vi "Determine Path Points.vi"(8 "error in (no error)":errorcluster, 11 "Tool Path in":refnum<class "Tool Path.lvclass">) -> (0 "error out":errorcluster, 2 "Points":T1[](array[typedef]), 3 "Tool Path out":refnum<class "Tool Path.lvclass">)   [LabVIEW 2019, in "Tool Path.lvclass"]
uses:
  Tool Path.lvclass
  Parse/PathCommands/Point.ctl
  Parse/ParsePaths/Path.lvclass/Path.ctl
  Settings/Path Settings/Path Settings.lvclass/Path Settings.ctl
  Parse/PathCommands/PathCommands.lvclass
  Parse/ParsePaths/Path.lvclass
  Settings/Path Settings/Path Settings.lvclass
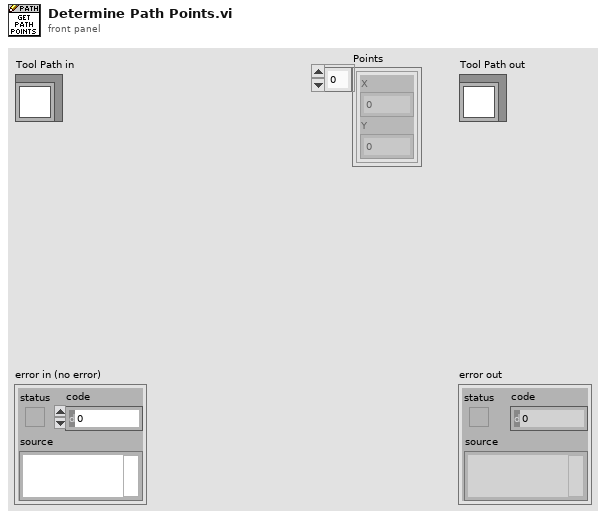
[diagram p1: front panel]
types:
  T1 = typedef "PathCommands.lvclass/Point.ctl" = cluster{"X":dbl, "Y":dbl}
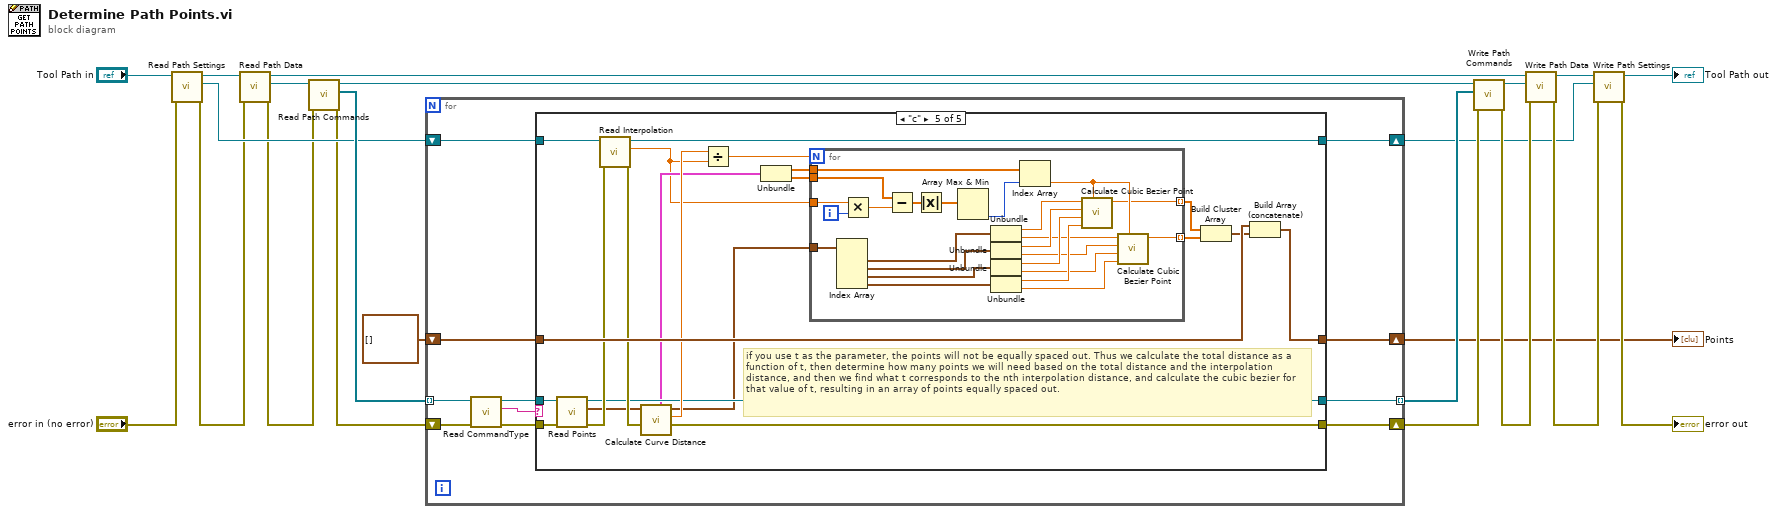
[diagram p0: block diagram]
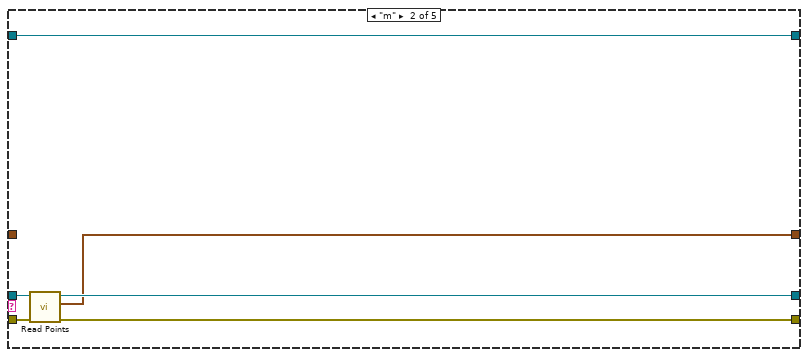
[diagram p3: hidden frame]
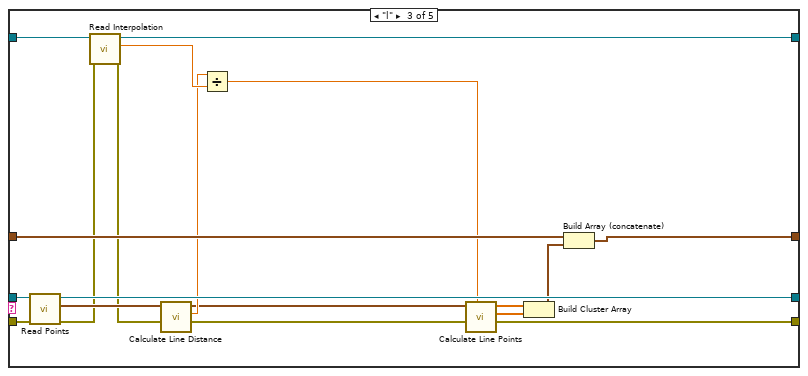
[diagram p4: hidden frame]
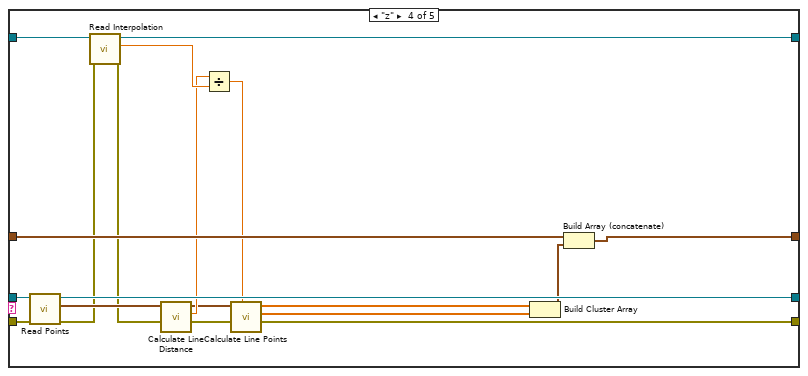
[diagram p5: hidden frame]
diagram:
  n1 = call-dynamic "Read Path Settings.vi"("error in (no error)"="error in (no error)", "Tool Path in"="Tool Path in") -> ("error out"=w11:errorcluster, "Path Settings.lvclass"=w13:refnum<class "Path Settings.lvclass">, "Tool Path out"=w17:refnum<class "Tool Path.lvclass">)  [unwired: 7 in]
  n2 = call-dynamic "Read Path Data.vi"("error in (no error)"=w11, "Tool Path in"=w17) -> ("error out"=w10:errorcluster, "Path.lvclass"=w16:refnum<class "Path.lvclass">, "Tool Path out"=w14:refnum<class "Tool Path.lvclass">)  [unwired: 7 in]
  n3 = call "Read Path Commands.vi"("error in (no error)"=w10, "Path in"=w16) -> ("error out"=w9:errorcluster, "Path Commands"=w21:refnum<class "PathCommands.lvclass">[], "Path out"=w22:refnum<class "Path.lvclass">)  [unwired: 7 in]
  n4 = for {
    shift-right: [w33] -> w7
    shift-left: w9 -> [w29]
    tunnel: w21 -> [w30] mode=indexing
    tunnel: [w32] -> w20 mode=indexing
    shift-right: [w23] -> w3
    shift-left: T1[] [] ("Points") -> [w26]
    shift-right: [w24] -> w2
    shift-left: w13 -> [w25]
    n5 = call-dynamic "Read CommandType.vi"("error in (no error)"=w29, "PathCommands in"=w30) -> ("error out"=w28:errorcluster, "CommandType"=w27:string, "PathCommands out"=w31:refnum<class "PathCommands.lvclass">)  [unwired: 7 in]
    n6 = case shown="\"c\"" w27 {
      tunnel: [w37 w41 w44 w67 w82] -> w33
      tunnel: w28 -> [w37 w40 w60 w79 w101]
      tunnel: [w36 w42 w61 w80 w93] -> w32
      tunnel: w31 -> [w36 w43 w62 w81 w102]
      tunnel: [w35 w38 w56 w75 w97] -> w23
      tunnel: w26 -> [w35 _ w55 w74 w98]
      tunnel: w25 -> [w34 w39 w58 w77 w99]
      tunnel: [w34 w39 w59 w78 w100] -> w24
      frame Default {
      }
      frame "m" {
        n7 = call-dynamic "Read Points.vi"("error in (no error)"=w40, "PathCommands in"=w43) -> ("error out"=w41:errorcluster, "Points"=w38:T1[], "PathCommands out"=w42:refnum<class "PathCommands.lvclass">)  [unwired: 7 in]
      }
      frame "l" {
        # "Create interpolation VI\nCreate Distance VI"
        n8 = call-dynamic "Read Points.vi"("error in (no error)"=w60, "PathCommands in"=w62) -> ("error out"=w47:errorcluster, "Points"=w54:T1[], "PathCommands out"=w61:refnum<class "PathCommands.lvclass">)  [unwired: 7 in]
        n9 = call "Read Interpolation.vi"("error in (no error)"=w47, "Path Settings in"=w58) -> ("error out"=w46:errorcluster, "Interpolation"=w57:dbl, "Path Settings out"=w59:refnum<class "Path Settings.lvclass">)  [unwired: 7 in]
        n10 = call "Calculate Line Distance.vi"("error in (no error)"=w46, "Points"=w54) -> ("error out"=w45:errorcluster, "Distance"=w53:dbl, "Points Out"=w52:T1[])  [unwired: 7 in]
        n11 = Divide(x=w53, y=w57) -> (x/y=w51:dbl)
        n12 = call "Calculate Line Points.vi"("Iterations"=w51, "error in (no error)"=w45, "Points"=w52) -> ("error out"=w44:errorcluster, "Y"=w50:dbl[], "X"=w49:dbl[])  [unwired: 6 in]
        n13 = Build Cluster Array(w49, w50) -> (w48:cluster{"X":dbl, "Y":dbl}[])
        n14 = Build Array (concatenate)(w55, w48) -> (w56:T1[])
      }
      frame "z" {
        # "Create interpolation VI\nCreate Distance VI"
        n15 = call-dynamic "Read Points.vi"("error in (no error)"=w79, "PathCommands in"=w81) -> ("error out"=w63:errorcluster, "Points"=w72:T1[], "PathCommands out"=w80:refnum<class "PathCommands.lvclass">)  [unwired: 7 in]
        n16 = call "Read Interpolation.vi"("error in (no error)"=w63, "Path Settings in"=w77) -> ("error out"=w64:errorcluster, "Interpolation"=w76:dbl, "Path Settings out"=w78:refnum<class "Path Settings.lvclass">)  [unwired: 7 in]
        n17 = call "Calculate Line Distance.vi"("error in (no error)"=w64, "Points"=w72) -> ("error out"=w68:errorcluster, "Distance"=w71:dbl, "Points Out"=w69:T1[])  [unwired: 7 in]
        n18 = Divide(x=w71, y=w76) -> (x/y=w70:dbl)
        n19 = call "Calculate Line Points.vi"("Iterations"=w70, "error in (no error)"=w68, "Points"=w69) -> ("error out"=w67:errorcluster, "Y"=w65:dbl[], "X"=w66:dbl[])  [unwired: 6 in]
        n20 = Build Cluster Array(w66, w65) -> (w73:cluster{"X":dbl, "Y":dbl}[])
        n21 = Build Array (concatenate)(w74, w73) -> (w75:T1[])
      }
      frame "c" {
        # "if you use t as the parameter, the points will not be equally spaced out. Thus we calculate the total distance as a function of t, then determine how many points we will need based on the total distance and the interpolation distance, and then we find what t corresponds to the nth interpolation distance, and calculate the cubic bezier for that value of t, resulting in an array of points equally spaced out."
        n22 = call-dynamic "Read Points.vi"("error in (no error)"=w101, "PathCommands in"=w102) -> ("error out"=w95:errorcluster, "Points"=w92:T1[], "PathCommands out"=w93:refnum<class "PathCommands.lvclass">)  [unwired: 7 in]
        n23 = call "Read Interpolation.vi"("error in (no error)"=w95, "Path Settings in"=w99) -> ("error out"=w94:errorcluster, "Interpolation"=w88:dbl, "Path Settings out"=w100:refnum<class "Path Settings.lvclass">)  [unwired: 7 in]
        n24 = call "Calculate Curve Distance.vi"("error in (no error)"=w94, "Points"=w92) -> ("error out"=w82:errorcluster, "Length"=w96:dbl, "Points Out"=w86:T1[], "Distance vs t"=w90:cluster{"t":dbl[], "Distance":dbl[]})  [unwired: 6 in]
        n25 = Divide(x=w96, y=w88) -> (x/y=w91:dbl)
        n26 = Unbundle(w90) -> ("t"=w87:dbl[], "Distance"=w89:dbl[])
        n27 = for {
          N: w91 -> [_]
          tunnel: w89 -> [w124]
          tunnel: w88 -> [w125]
          tunnel: w87 -> [w120]
          tunnel: w86 -> [w103]
          tunnel: [w105] -> w84 mode=indexing
          tunnel: [w104] -> w85 mode=indexing
          i -> [w126]
          n28 = Index Array(array=w103) -> (element #1=w110:T1, element #2=w109:T1, element #3=w108:T1, element #4=w107:T1)  [unwired: 4 in]
          n29 = Multiply(x=w125, y=w126) -> (x*y=w123:dbl)
          n30 = Subtract(x=w124, y=w123) -> (x-y=w122:dbl[])
          n31 = Absolute Value(x=w122) -> (abs(x)=w121:dbl[])
          n32 = Array Max & Min(array=w121) -> (min index (indices)=w119:i32)  [unwired: 3 out]
          n33 = Unbundle(w110) -> ("X"=w118:dbl, "Y"=w114:dbl)
          n34 = Unbundle(w109) -> ("X"=w115:dbl, "Y"=w113:dbl)
          n35 = Unbundle(w108) -> ("X"=w116:dbl, "Y"=w112:dbl)
          n36 = Unbundle(w107) -> ("X"=w117:dbl, "Y"=w111:dbl)
          n37 = Index Array(array=w120, index=w119) -> (element=w106:dbl)
          n38 = call "Calculate Cubic Bezier Point.vi"("t"=w106, "d"=w117, "c"=w116, "b"=w115, "a"=w118) -> ("f(t)"=w104:dbl)  [unwired: 6 in]
          n39 = call "Calculate Cubic Bezier Point.vi"("t"=w106, "d"=w111, "c"=w112, "b"=w113, "a"=w114) -> ("f(t)"=w105:dbl)  [unwired: 6 in]
        }
        n40 = Build Cluster Array(w85, w84) -> (w83:cluster{"f(t)":dbl, "f(t)":dbl}[])
        n41 = Build Array (concatenate)(w98, w83) -> (w97:T1[])
      }
    }
  }
  "Points" <- w3
  n42 = call "Write Path Commands.vi"("error in (no error)"=w7, "Path Commands"=w20, "Path in"=w22) -> ("error out"=w4:errorcluster, "Path out"=w15:refnum<class "Path.lvclass">)  [unwired: 7 in]
  n43 = call-dynamic "Write Path Data.vi"("error in (no error)"=w4, "Path.lvclass"=w15, "Tool Path in"=w14) -> ("error out"=w5:errorcluster, "Tool Path out"=w8:refnum<class "Tool Path.lvclass">)  [unwired: 7 in]
  n44 = call-dynamic "Write Path Settings.vi"("error in (no error)"=w5, "Path Settings.lvclass"=w2, "Tool Path in"=w8) -> ("error out"=→"error out":errorcluster, "Tool Path out"=→"Tool Path out":refnum<class "Tool Path.lvclass">)  [unwired: 7 in]
